vi "initFileContentsTree_NHMFL.vi"(4 "error in (no error)":errorcluster, 5 "file path":path, 6 "Tree Refnum":refnum<vi>, 7 "tdms file":refnum<k34>) -> (0 "error out":errorcluster, 3 "tdms file out":refnum<k34>)   [LabVIEW 2015]
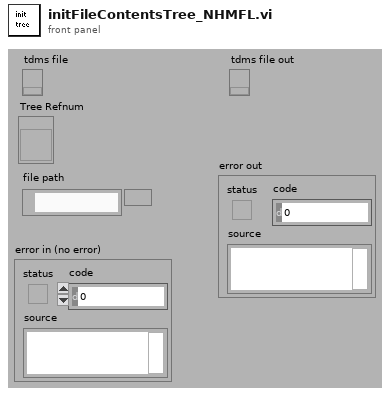
[diagram p1: front panel]
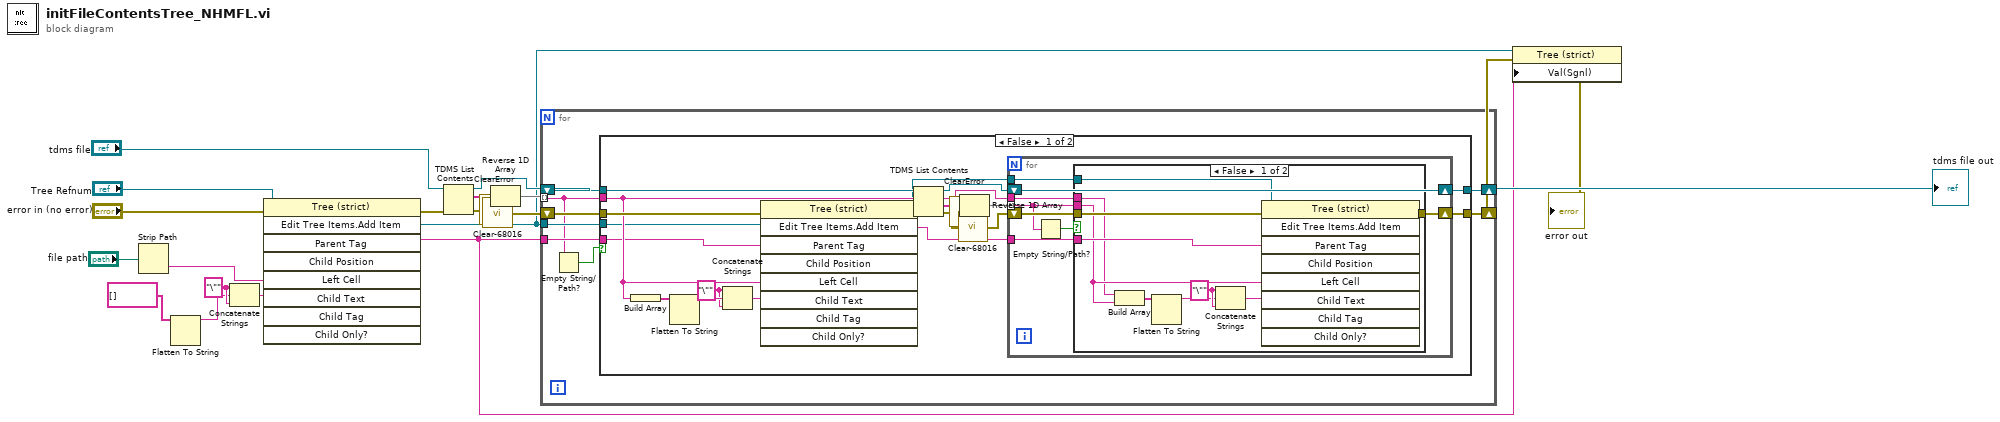
[diagram p0: block diagram]
diagram:
  w11 = "\"" ("string")
  n1 = Strip Path(path="file path") -> (name=w12:string)  [unwired: 1 out]
  n2 = Flatten To String(anything=string[] [] ("appended array")) -> (data string=w10:string)  [unwired: 3 in, 2 out]
  n3 = Concatenate Strings(w11, w10, w11) -> (w2:string)
  n4 = invoke on="Invoke Node" class="Tree (strict)" method="Edit Tree Items.Add Item"(reference="Tree Refnum", error in="error in (no error)", "Left Cell"=w12, "Child Tag"=w2) -> (reference out=w3:refnum<vi>, error out=w16:errorcluster, "Edit Tree Items:Add Item"=w1:string)  [unwired: 5 in, 6 out]
  n5 = TDMS List Contents(4:w16, 7:"tdms file") -> (0:w5:errorcluster, 2:w8:string[], 3:w17:refnum<k34>)  [unwired: 1 in, 1 out]
  n6 = call <vilib>:"ClearError.vi"("error in (no error)"=w5) -> ("error out"=w7:errorcluster)
  n7 = call <vilib>:"Clear-68016.vi"("error in (no error)"=w7) -> ("error out"=w6:errorcluster)
  n8 = Reverse 1D Array(array=w8) -> (reversed array=w19:string[])
  n9 = for {
    tunnel: w19 -> [w23] mode=indexing
    shift-right: [w26] -> w20
    shift-left: w17 -> [w28]
    shift-right: [w27] -> w21
    shift-left: w6 -> [w29]
    tunnel: w3 -> [w25]
    tunnel: w1 -> [w24]
    n10 = Empty String/Path?(string/path=w23) -> (empty?=w22:bool)
    n11 = case shown="False" w22 {
      tunnel: w29 -> [w50 w70]
      tunnel: w28 -> [w48 w71]
      tunnel: [w47 w70] -> w27
      tunnel: [w45 w71] -> w26
      tunnel: w23 -> [w43 _]
      tunnel: w25 -> [w36 _]
      tunnel: w24 -> [w34 _]
      frame False {
        w37 = "\"" ("string")
        n12 = Build Array(w43) -> (w42:string[])
        n13 = Flatten To String(anything=w42) -> (data string=w39:string)  [unwired: 3 in, 2 out]
        n14 = Concatenate Strings(w37, w39, w37) -> (w38:string)
        n15 = invoke on="Invoke Node" class="Tree (strict)" method="Edit Tree Items.Add Item"(reference=w36, error in=w50, "Parent Tag"=w34, "Left Cell"=w43, "Child Tag"=w38) -> (reference out=w35:refnum<vi>, error out=w49:errorcluster, "Edit Tree Items:Add Item"=w44:string)  [unwired: 4 in, 6 out]
        n16 = TDMS List Contents(4:w49, 6:w43, 7:w48) -> (0:w30:errorcluster, 1:w33:string[], 2:w41:string, 3:w46:refnum<k34>)
        n17 = call <vilib>:"ClearError.vi"("error in (no error)"=w30) -> ("error out"=w32:errorcluster)
        n18 = call <vilib>:"Clear-68016.vi"("error in (no error)"=w32) -> ("error out"=w31:errorcluster)
        n19 = Reverse 1D Array(array=w33) -> (reversed array=w40:string[])
        n20 = for {
          tunnel: w40 -> [w52] mode=indexing
          shift-right: [w56] -> w45
          shift-left: w46 -> [w56]
          shift-right: [w57] -> w47
          shift-left: w31 -> [w58]
          tunnel: w44 -> [w55]
          tunnel: w41 -> [w54]
          tunnel: w35 -> [w51]
          n21 = Empty String/Path?(string/path=w52) -> (empty?=w53:bool)
          n22 = case shown="False" w53 {
            tunnel: w58 -> [w68 w69]
            tunnel: [w67 w69] -> w57
            tunnel: w55 -> [w66 _]
            tunnel: w52 -> [w64 _]
            tunnel: w54 -> [w63 _]
            tunnel: w51 -> [w59 _]
            frame False {
              w62 = "\"" ("string")
              n23 = Build Array(w63, w64) -> (w65:string[])
              n24 = Flatten To String(anything=w65) -> (data string=w60:string)  [unwired: 3 in, 2 out]
              n25 = Concatenate Strings(w62, w60, w62) -> (w61:string)
              n26 = invoke on="Invoke Node" class="Tree (strict)" method="Edit Tree Items.Add Item"(reference=w59, error in=w68, "Parent Tag"=w66, "Left Cell"=w64, "Child Tag"=w61) -> (error out=w67:errorcluster)  [unwired: 4 in, 8 out]
            }
            frame True {
            }
          }
        }
      }
      frame True {
      }
    }
  }
  "tdms file out" <- w20
  n27 = property class="Tree (strict)"(reference=w3, error in=w21, "Val(Sgnl)"=w1) -> (error out=→"error out":errorcluster)  [unwired: 1 out]
